vi "Arm C Code (SubVI).vi"(6 "desiredAngle":dbl, 9 "initSpeed":dbl, 10 "potAngle":dbl, 11 "encoderHz":dbl) -> (3 "motorSpeed":dbl)   [LabVIEW 2015]
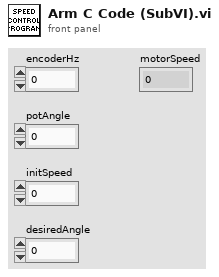
[diagram p1: front panel]
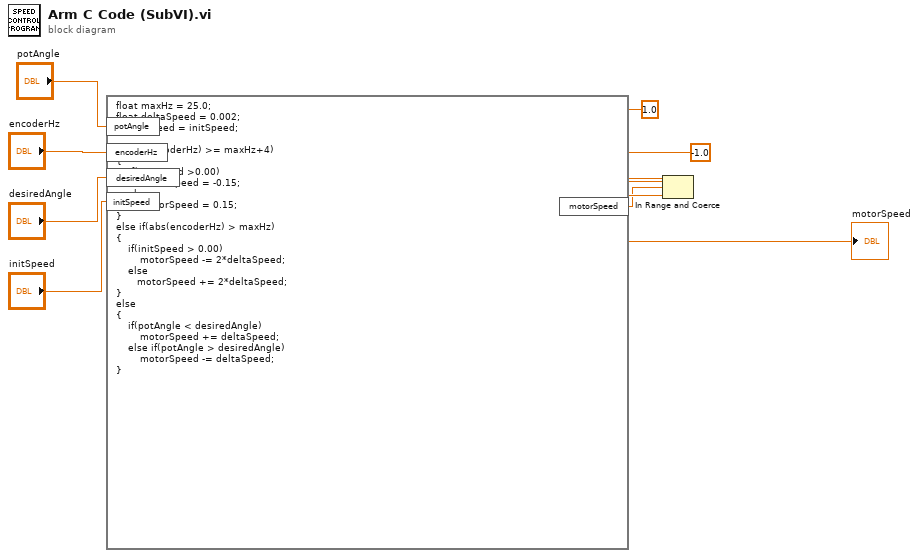
[diagram p0: block diagram]
diagram:
  n1 = formula code="float maxHz = 25.0;\nfloat deltaSpeed = 0.002;\nmotorSpeed = initSpeed;\n\nif(abs(encoderHz) >= maxHz+4)\n{\n    if(initSpeed >0.00)\n        motorSpeed = -0.15;\n    else\n        motorSpeed = 0.15;\n}\nelse if(abs(encoderHz) > maxHz)\n{\n    if(initSpeed > 0.00)\n        motorSpeed -= 2*deltaSpeed;\n    else\n       motorSpeed += 2*deltaSpeed;\n}\nelse\n{\n    if(potAngle < desiredAngle)\n        motorSpeed += deltaSpeed;\n    else if(potAngle > desiredAngle)\n        motorSpeed -= deltaSpeed;\n}"("potAngle"="potAngle", "encoderHz"="encoderHz", "desiredAngle"="desiredAngle", "initSpeed"="initSpeed") -> ("motorSpeed"=w1:dbl)
  n2 = In Range and Coerce(upper limit=1.0, x=w1, lower limit=-1.0) -> (coerced(x)=→"motorSpeed":dbl)  [unwired: 1 out]
